vi "obj_DataLog Mirror State.vi"(0 "method":T1, 5 "mirror in":T2, 7 "certificate in":string, 9 "db path in":path, 11 "local db":string, 12 "remote db in":string) -> (4 "present?":bool, 6 "mirror out":T2, 8 "certificate out":string, 10 "db path out":path, 14 "remote db out":string, 15 "get error":errorcluster)   [LabVIEW 2012]
doc: "Stores state required for mirroring. This state cannot be kept local to the mirror module instance since mirroring is also required when a flush of a tag in a mirrored database is requested before a query."
uses:
  typedefs/t_DataLog Mirror State Methods.ctl
  served/DataLog Mirror_srv.ctl
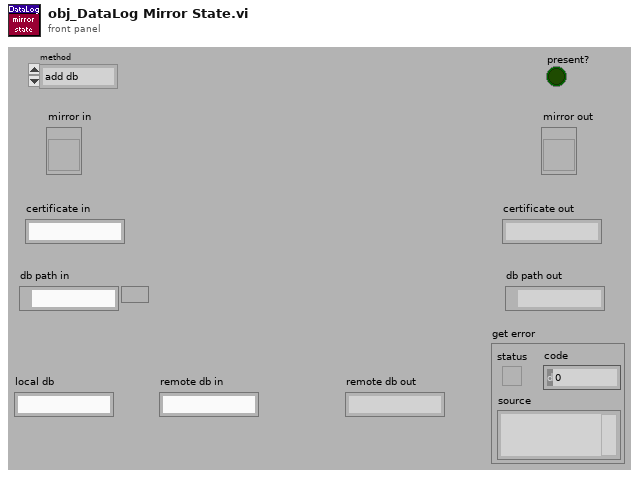
[diagram p1: front panel]
types:
  T1 = typedef "t_DataLog Mirror State Methods.ctl" = enum16{"add db", "check db", "set", "get", "unset", "clear"}
  T2 = typedef "DataLog Mirror_srv.ctl" = refnum<vi>
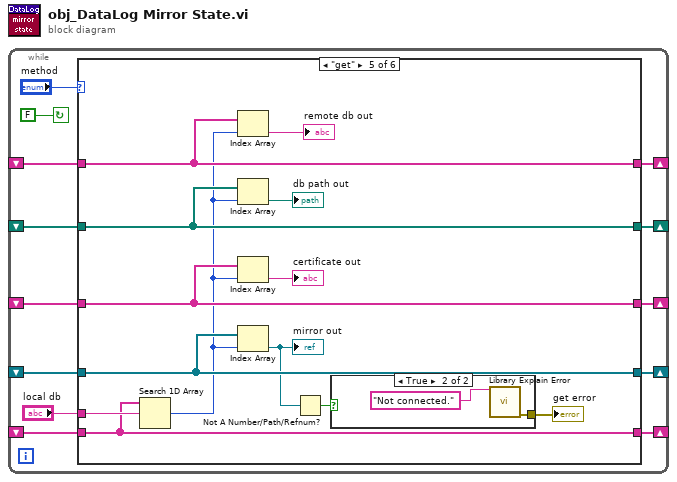
[diagram p0: block diagram]
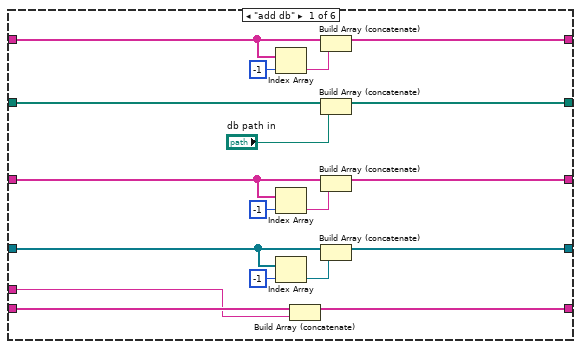
[diagram p2: hidden frame]
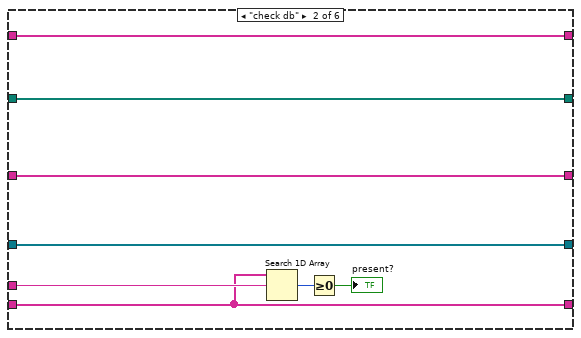
[diagram p3: hidden frame]
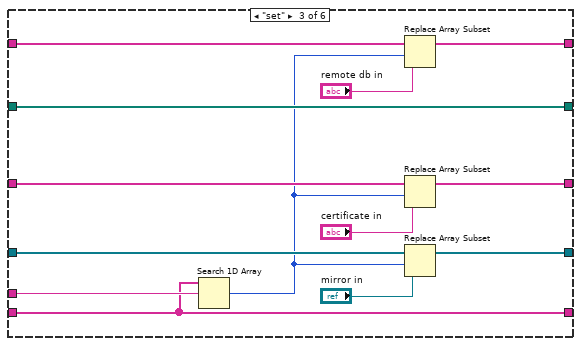
[diagram p4: hidden frame]
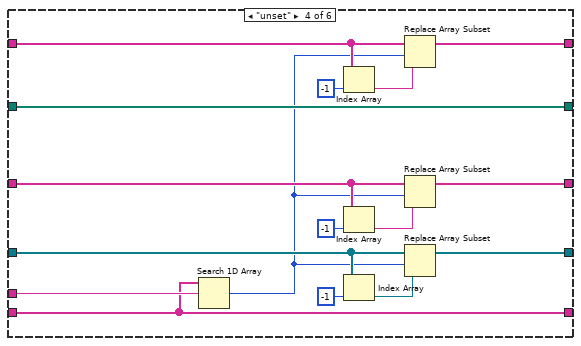
[diagram p5: hidden frame]
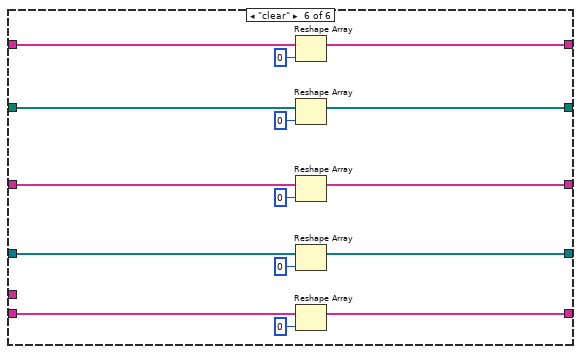
[diagram p7: hidden frame]
diagram:
  n1 = while {
    shift-right: [w11] -> _
    shift-left: _ -> [w12]
    shift-right: [w8] -> _
    shift-left: _ -> [w9]
    shift-right: [w5] -> _
    shift-left: _ -> [w6]
    shift-right: [w3] -> _
    shift-left: _ -> [w4]
    shift-right: [w1] -> _
    shift-left: _ -> [w2]
    stop <- FALSE continue-if-true
    n2 = case shown="\"get\"" "method" {
      tunnel: w12 -> [w29 w36 w50 w60 w79 w98]
      tunnel: [w28 w36 w48 w66 w79 w97] -> w11
      tunnel: w9 -> [w31 w37 w51 w67 w80 w95]
      tunnel: [w30 w37 w51 w67 w80 w93] -> w8
      tunnel: "local db" -> [w25 w38 w52 w68 w81 _]
      tunnel: w6 -> [w21 w34 w47 w64 w78 w92]
      tunnel: [w22 w34 w46 w65 w78 w90] -> w5
      tunnel: w4 -> [w20 w33 w44 w58 w76 w88]
      tunnel: [w19 w33 w44 w58 w76 w87] -> w3
      tunnel: [w14 w32 w42 w54 w74 w84] -> w1
      tunnel: w2 -> [w15 w32 w43 w55 w74 w85]
      frame "add db" {
        n3 = Index Array(array=w15, index=-1) -> (element=w17:string)
        n4 = Index Array(array=w21, index=-1) -> (element=w23:string)
        n5 = Index Array(array=w29, index=-1) -> (element=w27:T2)
        n6 = Build Array (concatenate)(w31, w25) -> (w30:string[])
        n7 = Build Array (concatenate)(w15, w17) -> (w14:string[])
        n8 = Build Array (concatenate)(w20, "db path in") -> (w19:path[])
        n9 = Build Array (concatenate)(w21, w23) -> (w22:string[])
        n10 = Build Array (concatenate)(w29, w27) -> (w28:T2[])
      }
      frame "check db" {
        n11 = Search 1D Array(1D array=w37, element=w38) -> (index of element=w39:i32)  [unwired: 1 in]
        n12 = Greater Or Equal To 0?(x=w39) -> (x >= 0?=→"present?":bool)
      }
      frame "set" {
        n13 = Search 1D Array(1D array=w51, element=w52) -> (index of element=w41:i32)  [unwired: 1 in]
        n14 = Replace Array Subset(array=w43, new element="remote db in", index=w41) -> (w42:string[])
        n15 = Replace Array Subset(array=w47, new element="certificate in", index=w41) -> (w46:string[])
        n16 = Replace Array Subset(array=w50, new element="mirror in", index=w41) -> (w48:T2[])
      }
      frame "unset" {
        n17 = Search 1D Array(1D array=w67, element=w68) -> (index of element=w53:i32)  [unwired: 1 in]
        n18 = Index Array(array=w55, index=-1) -> (element=w57:string)
        n19 = Index Array(array=w64, index=-1) -> (element=w62:string)
        n20 = Index Array(array=w60, index=-1) -> (element=w59:T2)
        n21 = Replace Array Subset(array=w55, new element=w57, index=w53) -> (w54:string[])
        n22 = Replace Array Subset(array=w64, new element=w62, index=w53) -> (w65:string[])
        n23 = Replace Array Subset(array=w60, new element=w59, index=w53) -> (w66:T2[])
      }
      frame "get" {
        n24 = Search 1D Array(1D array=w80, element=w81) -> (index of element=w72:i32)  [unwired: 1 in]
        n25 = Index Array(array=w74, index=w72) -> (element=→"remote db out":string)
        n26 = Index Array(array=w76, index=w72) -> (element=→"db path out":path)
        n27 = Index Array(array=w78, index=w72) -> (element=→"certificate out":string)
        n28 = Index Array(array=w79, index=w72) -> (element=w71:T2)
        "mirror out" <- w71
        n29 = Not A Number/Path/Refnum?(number/path/refnum=w71) -> (NaN/Path/Refnum?=w70:bool)
        n30 = case shown="True" w70 {
          tunnel: [_ w83] -> w69
          frame False {
          }
          frame True {
            n31 = call "Library Explain Error.vi"("explanation prefix (none)"="Not connected.") -> ("explained error"=w83:errorcluster)  [unwired: 14 in]
          }
        }
        "get error" <- w69
      }
      frame "clear" {
        n32 = Reshape Array(w85, 0 ("dimension size")) -> (w84:string[])
        n33 = Reshape Array(w88, 0 ("dimension size")) -> (w87:path[])
        n34 = Reshape Array(w92, 0 ("dimension size")) -> (w90:string[])
        n35 = Reshape Array(w98, 0 ("dimension size")) -> (w97:T2[])
        n36 = Reshape Array(w95, 0 ("dimension size")) -> (w93:string[])
      }
    }
  }
